vi "FGV_Camera.vi"(5 "File Path":path, 7 "action_camera":T3, 8 "error in":errorcluster, 10 "Image In":T1, 11 "Session In":T2) -> (0 "error out":errorcluster, 2 "Image Out":T1, 3 "Session Out":T2)   [LabVIEW 2015]
uses:
  <userlib>/FGV/control/Control_Camera.ctl
  <vilib>/userdefined/High Color/IMAQdx.ctl
  <vilib>/vision/Image Controls.llb/IMAQ Image.ctl
  <vilib>/vision/driver/NI_Vision_Acquisition_Software.lvlib
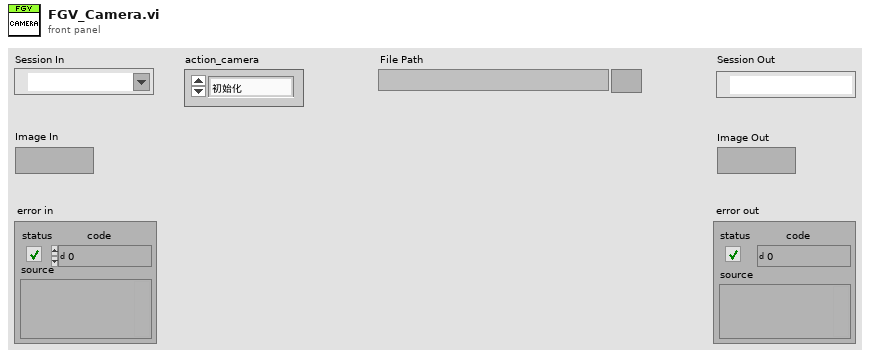
[diagram p1: front panel]
types:
  T1 = typedef "IMAQ Image.ctl" = refnum<image>
  T2 = typedef "IMAQdx.ctl" = refnum<k21>
  T3 = typedef "Control_Camera.ctl" = enum16{"初始化", "取像", "匯入影像", "結束"}
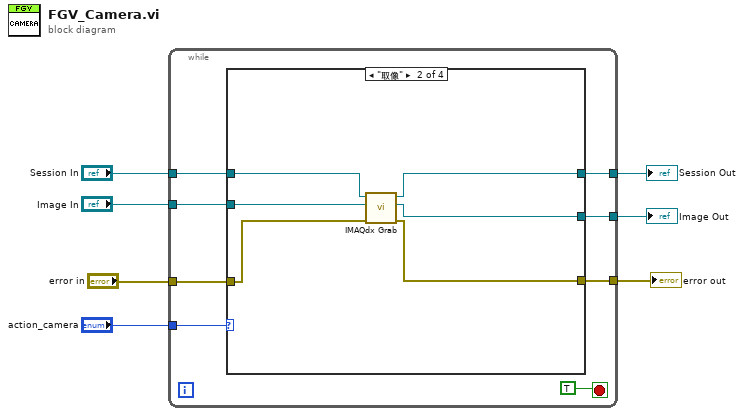
[diagram p0: block diagram]
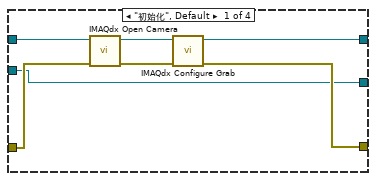
[diagram p2: hidden frame]
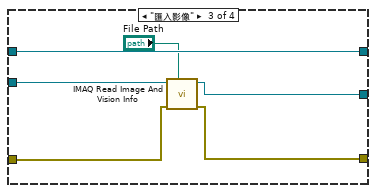
[diagram p3: hidden frame]
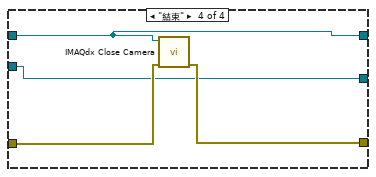
[diagram p4: hidden frame]
diagram:
  n1 = while {
    tunnel: "action_camera" -> [w14]
    tunnel: "Session In" -> [w13]
    tunnel: [w12] -> w5
    tunnel: "Image In" -> [w11]
    tunnel: [w10] -> w3
    tunnel: "error in" -> [w9]
    tunnel: [w8] -> w2
    stop <- TRUE stop-if-true
    n2 = case shown="\"取像\"" w14 {
      tunnel: w13 -> [w20 w23 w30 w35]
      tunnel: [w19 w28 w30 w35] -> w12
      tunnel: w11 -> [w16 w27 w34 w36]
      tunnel: [w16 w26 w33 w36] -> w10
      tunnel: w9 -> [w18 w25 w32 w37]
      tunnel: [w17 w24 w31 w38] -> w8
      frame "初始化", Default {
        n3 = call <vilib>:"IMAQdx Open Camera.vi"("error in"=w18, "Session In"=w20) -> ("error out"=w22:errorcluster, "Session Out"=w21:T2)  [unwired: 8 in]
        n4 = call <vilib>:"IMAQdx Configure Grab.vi"("error in"=w22, "Session In"=w21) -> ("error out"=w17:errorcluster, "Session Out"=w19:T2)  [unwired: 8 in]
      }
      frame "取像" {
        n5 = call <vilib>:"IMAQdx Grab.vi"("error in"=w25, "Image In"=w27, "Session In"=w23) -> ("error out"=w24:errorcluster, "Image Out"=w26:T1, "Session Out"=w28:T2)  [unwired: 5 in, 1 out]
      }
      frame "匯入影像" {
        n6 = call "IMAQ Read Image And Vision Info"("File Path"="File Path", "error in (no error)"=w32, "Image"=w34) -> ("error out"=w31:errorcluster, "Image Out"=w33:T1)  [unwired: 6 in, 1 out]
      }
      frame "結束" {
        n7 = call <vilib>:"IMAQdx Close Camera.vi"("error in"=w37, "Session In"=w35) -> ("error out"=w38:errorcluster)  [unwired: 9 in]
      }
    }
  }
  "Session Out" <- w5
  "Image Out" <- w3
  "error out" <- w2
